vi "Example Simple Voltage.vi"() -> ()   [LabVIEW 2013]
uses:
  C:/tf/play/labview/Tinkerforge.dll
  Tinkerforge.dll
panel:
  in  "uid":string="amb"
  in  "port":i32=4223
  in  "host":string="localhost"
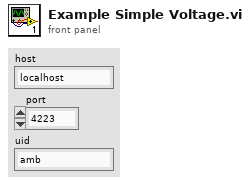
[diagram p1: front panel]
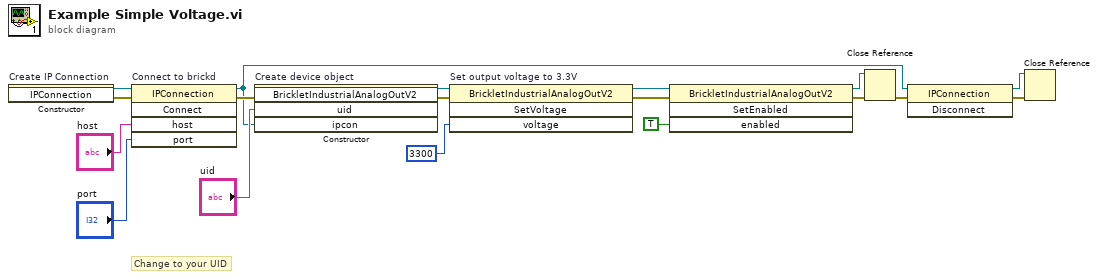
[diagram p0: block diagram]
diagram:
  # "Change to your UID"
  n1 = constructor on="Create IP Connection" class="IPConnection"() -> (reference out=w18:refnum<k24>, error out=w6:errorcluster)  [unwired: 3 in, 1 out]
  n2 = invoke on="Connect to brickd" class="IPConnection" method="Connect"(reference=w18, error in=w6, "host"="host", "port"="port") -> (reference out=w9:refnum<k24>, error out=w14:errorcluster)  [unwired: 1 in, 3 out]
  n3 = constructor on="Create device object" class="BrickletIndustrialAnalogOutV2"(error in=w14, "uid"="uid", "ipcon"=w9) -> (reference out=w12:refnum<k24>, error out=w13:errorcluster)  [unwired: 2 in, 3 out]
  n4 = invoke on="Set output voltage to 3.3V" class="BrickletIndustrialAnalogOutV2" method="SetVoltage"(reference=w12, error in=w13, "voltage"=3300) -> (reference out=w3:refnum<k24>, error out=w5:errorcluster)  [unwired: 1 in, 2 out]
  n5 = invoke class="BrickletIndustrialAnalogOutV2" method="SetEnabled"(reference=w3, error in=w5, "enabled"=TRUE) -> (reference out=w2:refnum<k24>, error out=w4:errorcluster)  [unwired: 1 in, 2 out]
  n6 = Close Reference(reference=w2, error in (no error)=w4) -> (error out=w11:errorcluster)
  n7 = invoke class="IPConnection" method="Disconnect"(reference=w9, error in=w11) -> (reference out=w8:refnum<k24>, error out=w10:errorcluster)  [unwired: 1 in, 1 out]
  n8 = Close Reference(reference=w8, error in (no error)=w10) -> ()  [unwired: 1 out]
